vi "NANOTEC-MOTORS.vi"() -> ()   [LabVIEW 2013]
uses:
  global_notaus.vi
  global_log_file.vi
panel:
  out "Bool Ref":T1
  in  "Tab Control":T2(tab)=enum."Standard Motor Operation"
  out "Created New Semaphor":bool
  in  "ComPort (VISA in)":refnum<visa-resource-name>="COM1"
  in  "ComConfig":T3={"Baudrate (115200)"=115200, "Data Bits (8)"=8, "Parity (None)"=0, "Stop Bits (1)"=10, "Flow Control (None)"=0, "End Mode for Reads (TermChar)"=2} {"End Mode for Reads (TermChar)" items=["None", "Last Bit", "TermChar"]; "Flow Control (None)" items=["None", "XON/XOFF", "RTS/CTS", "XON/XOFF & RTS/CTS", "DTR/DSR", "XON/XOFF & DTR/DSR"]; "Stop Bits (1)" items=["1.0"=10, "1.5"=15, "2.0"=20]; "Parity (None)" items=["None", "Odd", "Even", "Mark", "Space"]; "Baudrate (115200)" items=["115200"=115200, "19200"=19200]}
  in  "error in (no error)":errorcluster
  in  "Firmware":bool
  in  "Error Reset":bool
  out "Firmware 2":string
  out "error out":errorcluster
  out "VISA ressource out":refnum<visa-resource-name>
  out "Answer to Command":string
  in  "Command":string
  in  "Send Command":bool
  out "Current Position 2":string
  in  "Motor Adress 1":T4(ring)=enum."3" caption="Motor Adress"
  out "Answer Save Profile":string
  out "Answer V Start":string
  out "Answer Ramp":string
  out "Answer Break":string
  out "Answer Direction":string
  out "Answer Steps":string
  in  "Direction (d)":i32(ring) items=["left", "right"]
  in  "Steps (s)":u32=400
  out "Answer Operation Mode":string
  in  "V Start (u)":u32=1
  in  "V Normal (o)":u32=400
  in  "Ramp (b)":u32=10
  in  "Break (B)":u32=10
  in  "Save Profile":bool
  out "Answer V Normal":string
  in  "Number of Profile (>)":u32=1
  in  "Operation Mode (p)":u16(ring)=1 items=["Relative Positioning"=1, "Absolute Positioning"=2, "Internal Reference"=3, "External Reference"=4, "Speed"=5]
  in  "Save and Drive Profile":bool
  in  "Current Position":bool
  in  "Drive Profile":bool
  in  "Start Profile":bool
  in  "Stop Profile":bool
  out "Answer Stop":string
  out "Answer Start":string
  in  "Load Profile":bool
  out "Answer Load Profile":string
  in  "Read Current Profile":bool
  out "Answer Read Current Profile":string
  in  "Profile Nr.":i32=123456
  in  "Motor Adress 2":T4(ring)=enum."3" caption="Motor Adress"
  out "Delta Steps":i32
  in  "steps 0":bool
  in  "Refresh Log File":bool
  in  "steps 60000":bool
  in  "steps 48000":bool
  in  "steps 10000":bool
  in  "steps 5000":bool
  in  "steps 1000":bool
  in  "steps 500":bool
  in  "steps 50":bool
  in  "steps 100":bool
  in  "steps master":i32
  in  "Reload Standard Pr Para":bool
  in  "Notaus":bool
  out "Log File 2":string
  in  "Delete Log File 2":bool
  in  "exp cclock":bool
  in  "exp clock":bool
  in  "prep cclock":bool
  in  "prep clock":bool
  in  "right":bool
  in  "left":bool
  in  "down":bool
  in  "up":bool
  in  "in":bool
  in  "out":bool
  in  "Save Waypoint":bool
  in  "Delete Log File":bool
  out "Log File":string
  in  "Waypoints":u16(ring)=1 items=["WP 1 "=1, "WP 2"=2, "WP 3"=3, "WP 4"=4, "WP 5"=5]
  in  "Go to Waypoint":bool
  in  "Test WP function":bool
  in  "Reload Waypoint Profiles from Save File":bool
  in  "Reload Drivers Digital Input":bool
  in  "stop":bool
  # "(leave out # and \\r)"
  # "(\"?\" means Command is invalid)"
  # "(in Hz)"
  # "(in Hz)"
  # "(in Hz/ms)"
  # "(in Hz/ms)"
  # "[1-32]"
  # "STEPS"
  # "Standard Profile Parameters for Operation of Motors (V_Start, V_Stop, Ramp, Break, etc.)\nfor this Tab can be manipulated in the Code (Event-Structure Frame 20)."
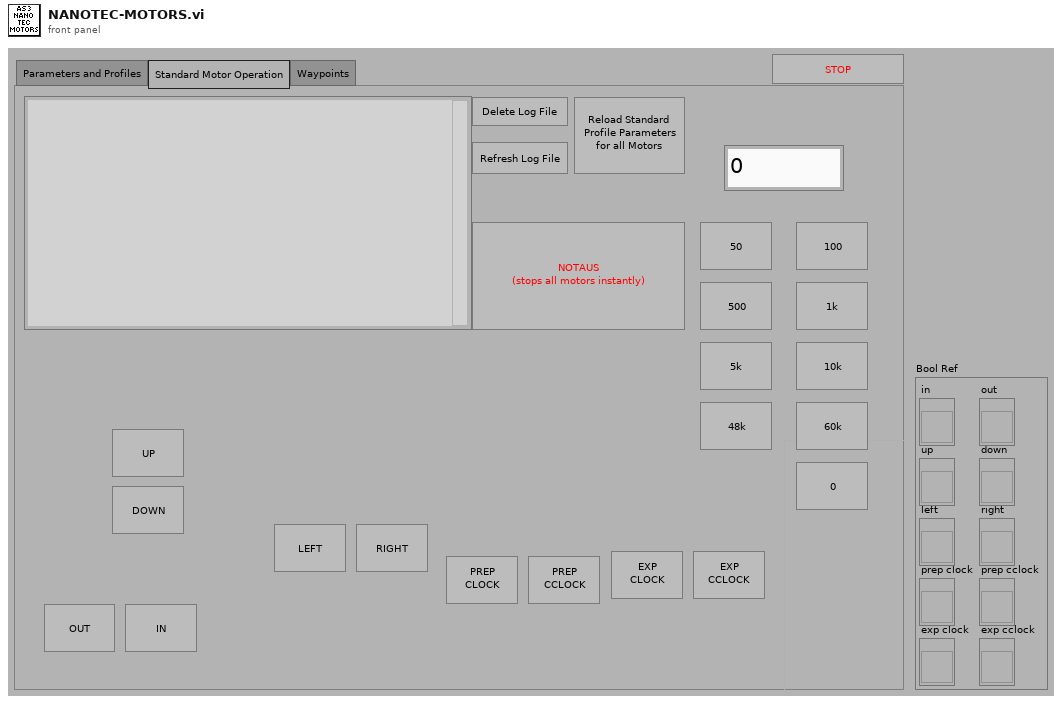
[diagram p1: front panel]
types:
  T1 = cluster{"in":refnum<vi>, "out":refnum<vi>, "up":refnum<vi>, "down":refnum<vi>, "left":refnum<vi>, "right":refnum<vi>, "prep clock":refnum<vi>, "prep cclock":refnum<vi>, "exp clock":refnum<vi>, "exp cclock":refnum<vi>}
  T2 = enum32{"Parameters and Profiles", "Standard Motor Operation", "Waypoints"}
  T3 = cluster{"Baudrate (115200)":u32, "Data Bits (8)":u16, "Parity (None)":u16, "Stop Bits (1)":u16, "Flow Control (None)":u16, "End Mode for Reads (TermChar)":u16}
  T4 = enum16{"All", "1", "2", "3", "4", "5", "6", "7", "8"}
  T5 = enum16{"open", "replace", "create", "open or create", "replace or create", "replace or create with confirmation"}
  T6 = typedef "Semaphore RefNum" = refnum<k1>
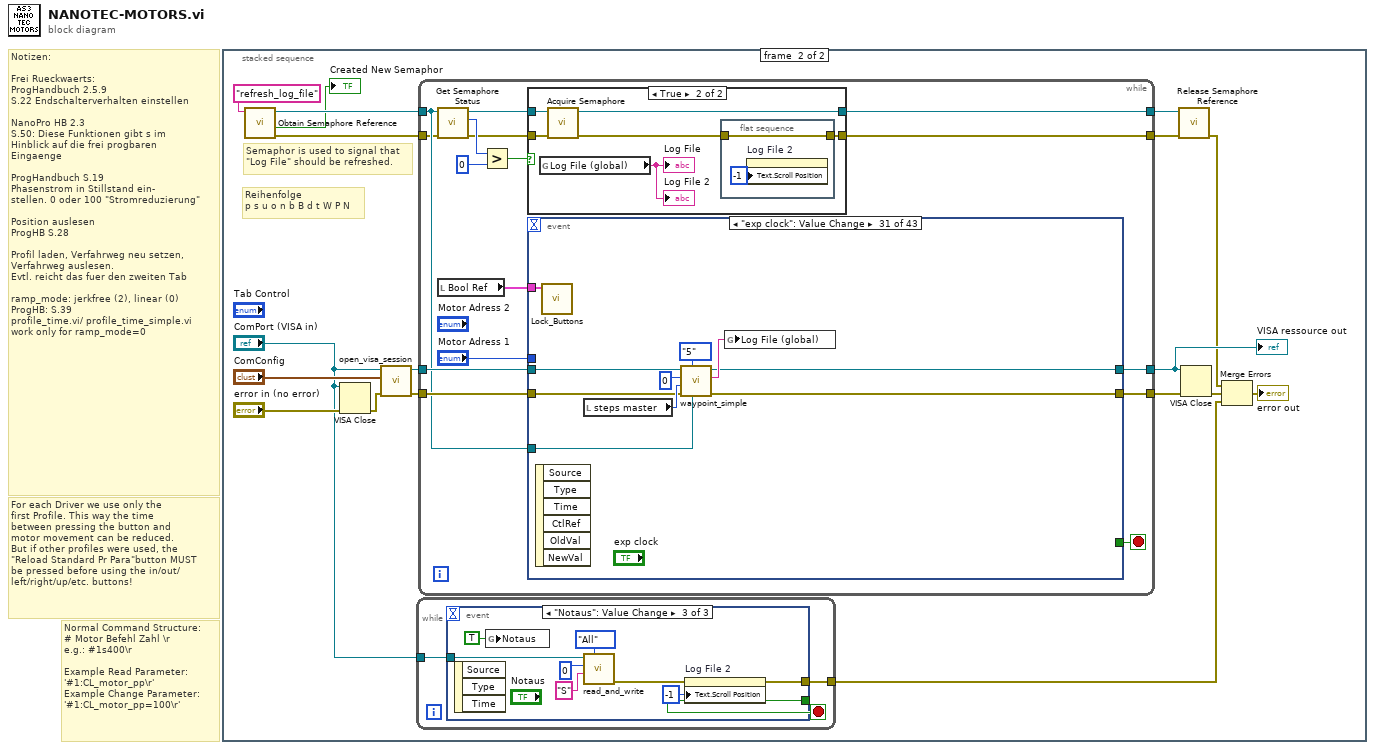
[diagram p0: block diagram]
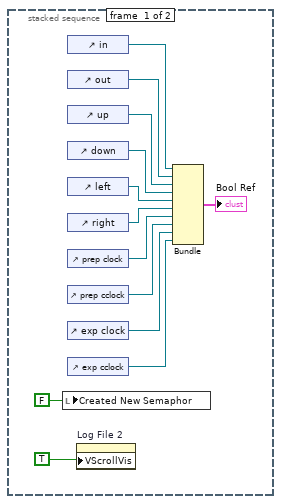
[diagram p2: hidden frame]
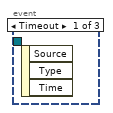
[diagram p3: hidden frame]
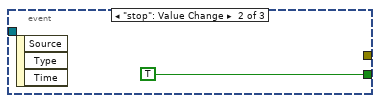
[diagram p4: hidden frame]
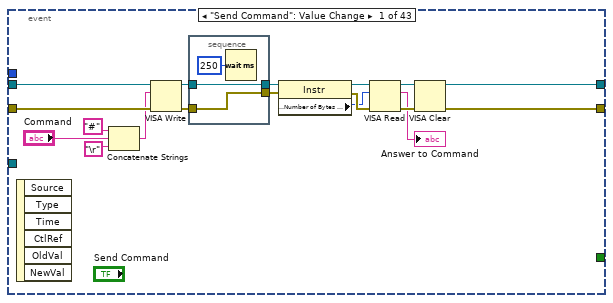
[diagram p6: hidden frame]
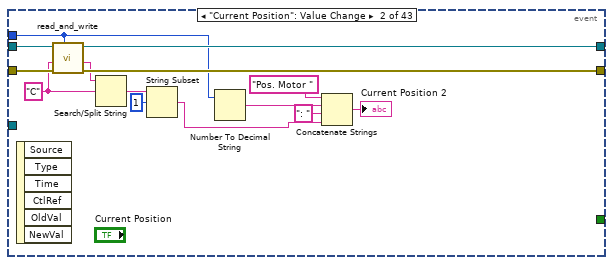
[diagram p7: hidden frame]
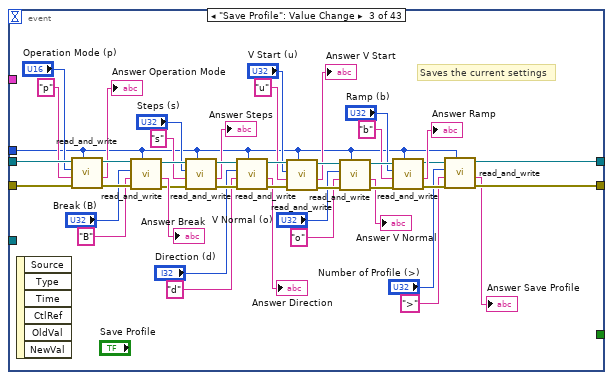
[diagram p8: hidden frame]
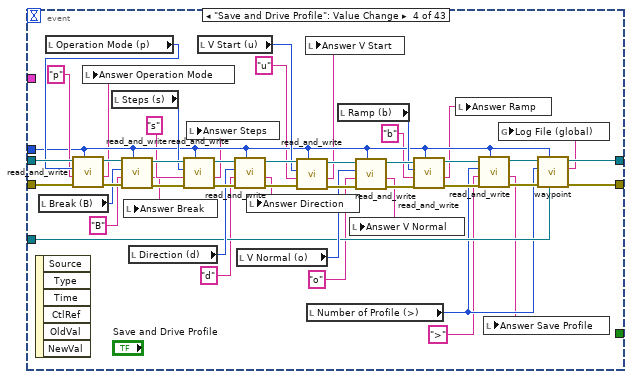
[diagram p9: hidden frame]
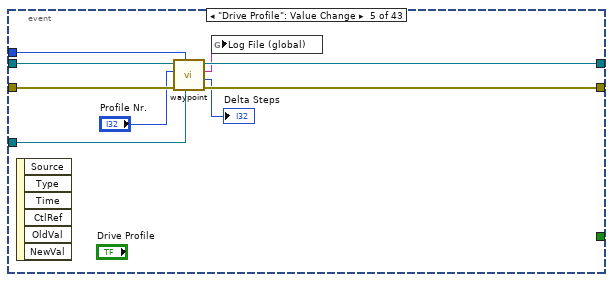
[diagram p10: hidden frame]
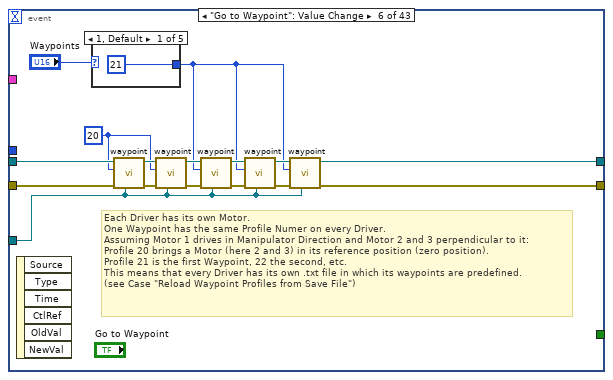
[diagram p11: hidden frame]
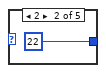
[diagram p12: hidden frame]
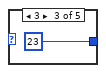
[diagram p13: hidden frame]
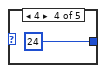
[diagram p14: hidden frame]
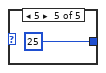
[diagram p15: hidden frame]
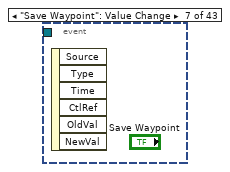
[diagram p16: hidden frame]
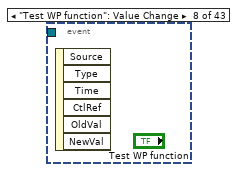
[diagram p17: hidden frame]
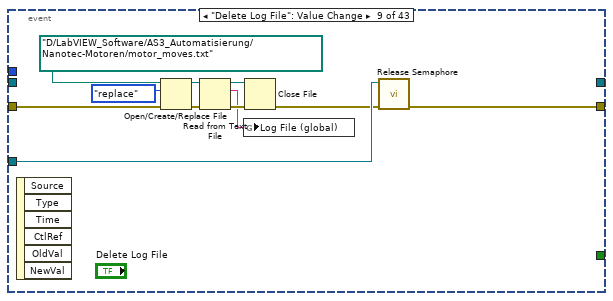
[diagram p18: hidden frame]
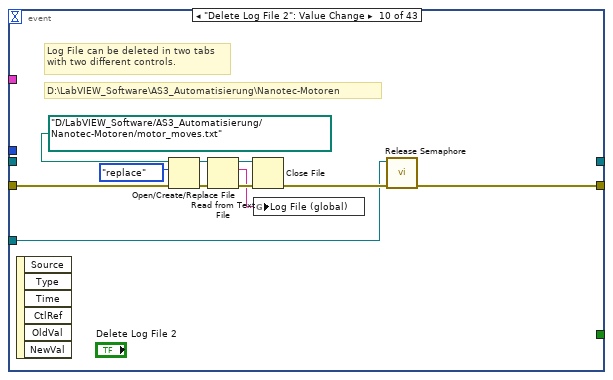
[diagram p19: hidden frame]
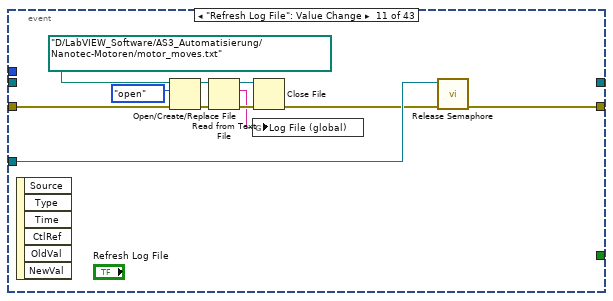
[diagram p20: hidden frame]
diagram:
  # "For each Driver we use only the\nfirst Profile. This way the time\nbetween pressing the button and\nmotor movement can be reduced.\nBut if other profiles were used, the\n\"Reload Standard Pr Para\"button MUST\nbe pressed before using the in/out/\nleft/right/up/etc. buttons!"
  # "Normal Command Structure:\n# Motor Befehl Zahl \\r\ne.g.: #1s400\\r\n\nExample Read Parameter:\n'#1:CL_motor_pp\\r'\nExample Change Parameter:\n'#1:CL_motor_pp=100\\r'"
  # "Notizen:\n\nFrei Rueckwaerts:\nProgHandbuch 2.5.9\nS.22 Endschalterverhalten einstellen\n\nNanoPro HB 2.3 \nS.50: Diese Funktionen gibt s im \nHinblick auf die frei progbaren \nEingaenge\n\nProgHandbuch S.19\nPhasenstrom in Stillstand ein-\nstellen. 0 oder 100 \"Stromreduzierung\"\n\nPosition auslesen\nProgHB S.28\n\nProfil laden, Verfahrweg neu setzen,\nVerfahrweg auslesen.\nEvtl. reicht das fuer den zweiten Tab\n\nramp_mode: jerkfree (2), linear (0) \nProgHB: S.39\nprofile_time.vi/ profile_time_simple.vi\nwork only for ramp_mode=0"
  n1 = stacked-sequence {
    frame #0 {
      n2 = local write "Created New Semaphor"(FALSE) -> ()
      n3 = control-ref of="in"() -> (w13:refnum<vi>)
      n4 = control-ref of="out"() -> (w12:refnum<vi>)
      n5 = control-ref of="up"() -> (w11:refnum<vi>)
      n6 = control-ref of="down"() -> (w10:refnum<vi>)
      n7 = control-ref of="left"() -> (w9:refnum<vi>)
      n8 = control-ref of="right"() -> (w8:refnum<vi>)
      n9 = control-ref of="prep clock"() -> (w7:refnum<vi>)
      n10 = control-ref of="prep cclock"() -> (w6:refnum<vi>)
      n11 = control-ref of="exp clock"() -> (w5:refnum<vi>)
      n12 = control-ref of="exp cclock"() -> (w4:refnum<vi>)
      n13 = property on="Log File 2" class="Str"("VScrollVis"=TRUE) -> ()  [unwired: 2 in, 2 out]
      n14 = Bundle("in"=w13, "out"=w12, "up"=w11, "down"=w10, "left"=w9, "right"=w8, "prep clock"=w7, "prep cclock"=w6, "exp clock"=w5, "exp cclock"=w4) -> (→"Bool Ref":T1)  [unwired: 1 in]
    }
    frame #1 {
      # "Reihenfolge\np s u o n b B d t W P N"
      # "Semaphor is used to signal that\n\"Log File\" should be refreshed."
      n15 = call <vilib>:"Obtain Semaphore Reference.vi"("name (unnamed)"="refresh_log_file") -> ("error out"=w21:errorcluster, "created new"=→"Created New Semaphor":bool, "semaphore"=w23:T6)  [unwired: 4 in]
      n16 = VISA Close(VISA resource name="ComPort (VISA in)", error in (no error)="error in (no error)") -> (error out=w27:errorcluster)
      n17 = call "open_visa_session.vi"("error in (no error)"=w27, "Cluster"="ComConfig", "ComPort"="ComPort (VISA in)") -> ("error out"=w30:errorcluster, "VISA resource name out"=w31:refnum<visa-resource-name>)  [unwired: 7 in]
      n18 = while {
        tunnel: "ComPort (VISA in)" -> [w33]
        tunnel: [w32] -> w14
        stop <- w34 stop-if-true
        n19 = event shown="[2] \"Notaus\": Value Change" {
          selector: _ -> [_ _ _]
          dyn-events: _ -> [_ _ _]
          timeout: _ -> [_ _ _]
          tunnel: [_ TRUE _] -> w34
          tunnel: w33 -> [_ _ w40]
          tunnel: [_ _ w36] -> w32
          event Timeout {
            n20 = event-data() -> ()  [unwired: 1 in, 3 out]
          }
          event "stop": Value Change {
            n21 = event-data() -> ()  [unwired: 1 in, 3 out]
          }
          event "Notaus": Value Change {
            n22 = event-data() -> ()  [unwired: 1 in, 3 out]
            n23 = global write "global_notaus.vi" "Notaus"(TRUE) -> ()
            n24 = call "read_and_write.vi"("Motor Adress"=T4."All", "Command"="S", "value"=0, "VISA ressource in"=w40) -> ("error out"=w37:errorcluster)  [unwired: 4 in, 3 out]
            n25 = property on="Log File 2" class="Str"(error in=w37, "Text.Scroll Position"=-1) -> (error out=w36:errorcluster)  [unwired: 1 in, 1 out]
          }
        }
      }
      n26 = while {
        tunnel: w31 -> [w59]
        tunnel: w30 -> [w58]
        tunnel: [w45] -> w29
        tunnel: [w57] -> w28
        tunnel: w23 -> [w50]
        tunnel: [w51] -> w22
        tunnel: w21 -> [w49]
        tunnel: [w47] -> w20
        stop <- w46 stop-if-true
        n27 = call <vilib>:"Get Semaphore Status.vi"("error in (no error)"=w49, "semaphore"=w50) -> ("error out"=w48:errorcluster, "# available"=w55:i32, "semaphore out"=w52:T6)  [unwired: 4 in, 3 out]
        n28 = local read "Bool Ref"() -> (w44:T1)
        n29 = Greater?(x=w55, y=0) -> (0:w53:bool)
        n30 = case shown="True" w53 {
          tunnel: w52 -> [w61 w67]
          tunnel: [w61 w66] -> w51
          tunnel: w48 -> [w60 w65]
          tunnel: [w60 w62] -> w47
          frame False {
          }
          frame True {
            n31 = global read "global_log_file.vi" "Log File (global)"() -> (→"Log File" →"Log File 2":string)
            n32 = call <vilib>:"Acquire Semaphore.vi"("error in (no error)"=w65, "semaphore"=w67) -> ("error out"=w63:errorcluster, "semaphore out"=w66:T6)  [unwired: 3 in, 1 out]
            n33 = flat-sequence {
              tunnel: w63 -> [w69]
              tunnel: [w69] -> w62
              frame #0 {
                n34 = property on="Log File 2" class="Str"("Text.Scroll Position"=-1) -> ()  [unwired: 2 in, 2 out]
              }
            }
          }
        }
        n35 = event shown="[30] \"exp clock\": Value Change" {
          selector: _ -> [_ _ _ _ _ _ _ _ _ _ _ _ _ _ _ _ _ _ _ _ _ _ _ _ _ _ _ _ _ _ _ _ _ _ _ _ _ _ _ _ _ _ _]
          dyn-events: _ -> [_ _ _ _ _ _ _ _ _ _ _ _ _ _ _ _ _ _ _ _ _ _ _ _ _ _ _ _ _ _ _ _ _ _ _ _ _ _ _ _ _ _ _]
          timeout: _ -> [_ _ _ _ _ _ _ _ _ _ _ _ _ _ _ _ _ _ _ _ _ _ _ _ _ _ _ _ _ _ _ _ _ _ _ _ _ _ _ _ _ _ _]
          tunnel: w59 -> [w78 w101 w146 w179 w203 w211 _ _ _ _ _ w265 w273 w281 w289 w294 w523 w575 w581 _ _ w587 w635 w643 w659 w669 w679 w689 w699 w709 w719 w729 _ _ _ _ _ _ _ _ _ _ _]
          tunnel: w58 -> [w77 w104 w147 w180 w202 w208 _ _ w232 w239 w249 w264 w272 w280 w288 w293 w521 w574 w580 _ _ w588 w633 w644 w653 w663 w673 w683 w693 w703 w713 w723 _ _ _ _ _ _ _ _ _ _ _]
          tunnel: [w76 w102 w124 w168 w201 w214 _ _ _ _ _ w261 w270 w279 w287 w291 w527 w572 w578 _ _ w585 w640 w647 w656 w666 w676 w686 w696 w706 w716 w726 _ _ _ _ _ _ _ _ _ _ _] -> w57
          tunnel: [w75 w103 w125 w166 w200 w215 _ _ w233 w237 w247 w260 w269 w278 w286 w292 w528 w571 w577 _ _ w586 w639 w648 w657 w667 w677 w687 w697 w707 w717 w727 _ _ _ _ _ _ _ _ _ _ _] -> w45
          tunnel: "Motor Adress 1" -> [_ w96 w105 w163 w199 _ _ _ _ _ _ w259 w267 w276 w283 w295 _ w569 w576 _ _ _ _ _ _ _ _ _ _ _ _ _ _ _ _ _ _ _ _ _ _ _ _]
          tunnel: w50 -> [_ _ _ w165 w197 w206 _ _ w234 w238 w257 _ _ w274 _ _ _ _ _ _ _ _ w637 w649 w658 w668 w678 w688 w698 w708 w718 w728 _ _ _ _ _ _ _ _ _ _ _]
          tunnel: [_ _ _ _ _ _ _ _ _ _ _ _ _ _ _ _ _ _ _ _ _ _ _ _ _ _ _ _ _ _ _ _ _ _ _ _ _ _ _ _ _ TRUE _] -> w46
          tunnel: w44 -> [_ _ _ _ _ _ _ _ _ _ _ _ _ _ _ _ _ _ _ _ _ _ w634 w645 w654 w664 w674 w684 w694 w704 w714 w724 _ _ _ _ _ _ _ _ _ _ _]
          event "Send Command": Value Change {
            n36 = event-data() -> ()  [unwired: 1 in, 6 out]
            n37 = Concatenate Strings("#" ("staticText"), "Command", "\r") -> (w72:string)
            n38 = VISA Write(VISA resource name=w78, write buffer=w72, error in (no error)=w77) -> (VISA resource name out=w82:refnum<visa-resource-name>, error out=w80:errorcluster)  [unwired: 1 out]
            n39 = stacked-sequence {
              tunnel: w82 -> [w90]
              tunnel: [w90] -> w81
              tunnel: w80 -> [w89]
              tunnel: [w89] -> w79
              frame #0 {
                n40 = Wait (ms)(milliseconds to wait=u32 250) -> ()  [unwired: 1 out]
              }
            }
            n41 = property class="Instr"(reference=w81, error in=w79) -> (reference out=w84:refnum<visa-resource-name>, error out=w85:errorcluster, "Serial Settings:Number of Bytes at Serial Port"=w83:u32)
            n42 = VISA Read(VISA resource name=w84, byte count=w83, error in (no error)=w85) -> (VISA resource name out=w87:refnum<visa-resource-name>, read buffer=→"Answer to Command":string, error out=w86:errorcluster)  [unwired: 1 out]
            n43 = VISA Clear(VISA resource name=w87, error in (no error)=w86) -> (VISA resource name out=w76:refnum<visa-resource-name>, error out=w75:errorcluster)
          }
          event "Current Position": Value Change {
            w99 = "C" ("Command")
            n44 = event-data() -> ()  [unwired: 1 in, 6 out]
            n45 = call "read_and_write.vi"("Motor Adress"=w96, "error in (no error)"=w104, "Command"=w99, "VISA ressource in"=w101) -> ("error out"=w103:errorcluster, "Answer"=w100:string, "VISA ressource out"=w102:refnum<visa-resource-name>)  [unwired: 4 in, 1 out]
            n46 = Search/Split String(string=w100, search string/char (-)=w99) -> (match + rest of string=w98:string)  [unwired: 1 in, 2 out]
            n47 = String Subset(string=w98, offset (0)=1) -> (substring=w91:string)  [unwired: 1 in]
            n48 = Number To Decimal String(number=w96) -> (decimal integer string=w94:string)  [unwired: 1 in]
            n49 = Concatenate Strings("Pos. Motor " ("string"), w94, ": " ("string"), w91) -> (→"Current Position 2":string)
          }
          event "Save Profile": Value Change {
            # "Saves the current settings"
            n50 = event-data() -> ()  [unwired: 1 in, 6 out]
            n51 = call "read_and_write.vi"("Motor Adress"=w105, "error in (no error)"=w147, "Command"="p" ("string"), "value"="Operation Mode (p)", "VISA ressource in"=w146) -> ("error out"=w144:errorcluster, "Answer"=→"Answer Operation Mode":string, "VISA ressource out"=w145:refnum<visa-resource-name>)  [unwired: 3 in, 1 out]
            n52 = call "read_and_write.vi"("Motor Adress"=w105, "error in (no error)"=w144, "Command"="B" ("command letter"), "value"="Break (B)", "VISA ressource in"=w145) -> ("error out"=w140:errorcluster, "Answer"=→"Answer Break":string, "VISA ressource out"=w141:refnum<visa-resource-name>)  [unwired: 3 in, 1 out]
            n53 = call "read_and_write.vi"("Motor Adress"=w105, "error in (no error)"=w140, "Command"="s" ("string"), "value"="Steps (s)", "VISA ressource in"=w141) -> ("error out"=w138:errorcluster, "Answer"=→"Answer Steps":string, "VISA ressource out"=w139:refnum<visa-resource-name>)  [unwired: 3 in, 1 out]
            n54 = call "read_and_write.vi"("Motor Adress"=w105, "error in (no error)"=w138, "Command"="d" ("string"), "value"="Direction (d)", "VISA ressource in"=w139) -> ("error out"=w136:errorcluster, "Answer"=→"Answer Direction":string, "VISA ressource out"=w137:refnum<visa-resource-name>)  [unwired: 3 in, 1 out]
            n55 = call "read_and_write.vi"("Motor Adress"=w105, "error in (no error)"=w136, "Command"="u" ("command letter"), "value"="V Start (u)", "VISA ressource in"=w137) -> ("error out"=w134:errorcluster, "Answer"=→"Answer V Start":string, "VISA ressource out"=w135:refnum<visa-resource-name>)  [unwired: 3 in, 1 out]
            n56 = call "read_and_write.vi"("Motor Adress"=w105, "error in (no error)"=w134, "Command"="o" ("command letter"), "value"="V Normal (o)", "VISA ressource in"=w135) -> ("error out"=w131:errorcluster, "Answer"=→"Answer V Normal":string, "VISA ressource out"=w129:refnum<visa-resource-name>)  [unwired: 3 in, 1 out]
            n57 = call "read_and_write.vi"("Motor Adress"=w105, "error in (no error)"=w131, "Command"="b" ("command letter"), "value"="Ramp (b)", "VISA ressource in"=w129) -> ("error out"=w127:errorcluster, "Answer"=→"Answer Ramp":string, "VISA ressource out"=w126:refnum<visa-resource-name>)  [unwired: 3 in, 1 out]
            n58 = call "read_and_write.vi"("Motor Adress"=w105, "error in (no error)"=w127, "Command"=">", "value"="Number of Profile (>)", "VISA ressource in"=w126) -> ("error out"=w125:errorcluster, "Answer"=→"Answer Save Profile":string, "VISA ressource out"=w124:refnum<visa-resource-name>)  [unwired: 3 in, 1 out]
          }
          event "Save and Drive Profile": Value Change {
            n59 = event-data() -> ()  [unwired: 1 in, 6 out]
            n60 = local read "Break (B)"() -> (w176:u32)
            n61 = local read "Operation Mode (p)"() -> (w178:u16)
            n62 = call "read_and_write.vi"("Motor Adress"=w163, "error in (no error)"=w180, "Command"="p", "value"=w178, "VISA ressource in"=w179) -> ("error out"=w193:errorcluster, "Answer"=w156:string, "VISA ressource out"=w194:refnum<visa-resource-name>)  [unwired: 3 in, 1 out]
            n63 = local write "Answer Operation Mode"(w156) -> ()
            n64 = local read "Steps (s)"() -> (w174:u32)
            n65 = call "read_and_write.vi"("Motor Adress"=w163, "error in (no error)"=w193, "Command"="B", "value"=w176, "VISA ressource in"=w194) -> ("error out"=w191:errorcluster, "Answer"=w155:string, "VISA ressource out"=w192:refnum<visa-resource-name>)  [unwired: 3 in, 1 out]
            n66 = local write "Answer Break"(w155) -> ()
            n67 = local read "Direction (d)"() -> (w173:i32)
            n68 = call "read_and_write.vi"("Motor Adress"=w163, "error in (no error)"=w191, "Command"="s", "value"=w174, "VISA ressource in"=w192) -> ("error out"=w189:errorcluster, "Answer"=w154:string, "VISA ressource out"=w190:refnum<visa-resource-name>)  [unwired: 3 in, 1 out]
            n69 = local write "Answer Steps"(w154) -> ()
            n70 = local read "V Start (u)"() -> (w172:u32)
            n71 = call "read_and_write.vi"("Motor Adress"=w163, "error in (no error)"=w189, "Command"="d", "value"=w173, "VISA ressource in"=w190) -> ("error out"=w187:errorcluster, "Answer"=w153:string, "VISA ressource out"=w188:refnum<visa-resource-name>)  [unwired: 3 in, 1 out]
            n72 = local read "V Normal (o)"() -> (w171:u32)
            n73 = local write "Answer Direction"(w153) -> ()
            n74 = call "read_and_write.vi"("Motor Adress"=w163, "error in (no error)"=w187, "Command"="u", "value"=w172, "VISA ressource in"=w188) -> ("error out"=w185:errorcluster, "Answer"=w152:string, "VISA ressource out"=w186:refnum<visa-resource-name>)  [unwired: 3 in, 1 out]
            n75 = local write "Answer V Start"(w152) -> ()
            n76 = local read "Number of Profile (>)"() -> (w164:u32)
            n77 = local read "Ramp (b)"() -> (w170:u32)
            n78 = call "read_and_write.vi"("Motor Adress"=w163, "error in (no error)"=w185, "Command"="o", "value"=w171, "VISA ressource in"=w186) -> ("error out"=w184:errorcluster, "Answer"=w151:string, "VISA ressource out"=w183:refnum<visa-resource-name>)  [unwired: 3 in, 1 out]
            n79 = local write "Answer V Normal"(w151) -> ()
            n80 = call "read_and_write.vi"("Motor Adress"=w163, "error in (no error)"=w184, "Command"="b", "value"=w170, "VISA ressource in"=w183) -> ("error out"=w182:errorcluster, "Answer"=w150:string, "VISA ressource out"=w181:refnum<visa-resource-name>)  [unwired: 3 in, 1 out]
            n81 = local write "Answer Ramp"(w150) -> ()
            n82 = call "read_and_write.vi"("Motor Adress"=w163, "error in (no error)"=w182, "Command"=">", "value"=w164, "VISA ressource in"=w181) -> ("error out"=w167:errorcluster, "Answer"=w149:string, "VISA ressource out"=w169:refnum<visa-resource-name>)  [unwired: 3 in, 1 out]
            n83 = local write "Answer Save Profile"(w149) -> ()
            n84 = call "waypoint.vi"("semaphore"=w165, "Motor Adress"=w163, "error in (no error)"=w167, "Profile Number"=w164, "VISA ressource in"=w169) -> ("error out"=w166:errorcluster, "Log File"=w148:string, "VISA ressource out"=w168:refnum<visa-resource-name>)  [unwired: 3 in, 1 out]
            n85 = global write "global_log_file.vi" "Log File (global)"(w148) -> ()
          }
          event "Drive Profile": Value Change {
            n86 = event-data() -> ()  [unwired: 1 in, 6 out]
            n87 = call "waypoint.vi"("semaphore"=w197, "Motor Adress"=w199, "error in (no error)"=w202, "Profile Number"="Profile Nr.", "VISA ressource in"=w203) -> ("error out"=w200:errorcluster, "Delta Steps"=→"Delta Steps":i32, "Log File"=w198:string, "VISA ressource out"=w201:refnum<visa-resource-name>)  [unwired: 3 in]
            n88 = global write "global_log_file.vi" "Log File (global)"(w198) -> ()
          }
          event "Go to Waypoint": Value Change {
            w204 = 20 ("Profile Number")
            # "Each Driver has its own Motor.\nOne Waypoint has the same Profile Numer on every Driver.\nAssuming Motor 1 drives in Manipulator Direction and Motor 2 and 3 perpendicular to it:\nProfile 20 brings a Motor (here 2 and 3) in its reference position (zero position).\nProfile 21 is the first Waypoint, 22 the second, etc.\nThis means that every Driver has its own .txt file in which its waypoints are predefined.\n(see Case \"Reload Waypoint Profiles from Save File\")"
            n89 = event-data() -> ()  [unwired: 1 in, 6 out]
            n90 = case shown="1, Default" "Waypoints" {
              tunnel: [21 22 23 24 25] -> w205
              frame 1, Default {
              }
              frame 2 {
              }
              frame 3 {
              }
              frame 4 {
              }
              frame 5 {
              }
            }
            n91 = call "waypoint.vi"("semaphore"=w206, "error in (no error)"=w208, "Profile Number"=w204, "VISA ressource in"=w211) -> ("error out"=w209:errorcluster, "VISA ressource out"=w212:refnum<visa-resource-name>)  [unwired: 4 in, 2 out]
            n92 = call "waypoint.vi"("semaphore"=w206, "error in (no error)"=w209, "Profile Number"=w204, "VISA ressource in"=w212) -> ("error out"=w207:errorcluster, "VISA ressource out"=w210:refnum<visa-resource-name>)  [unwired: 4 in, 2 out]
            n93 = call "waypoint.vi"("semaphore"=w206, "error in (no error)"=w207, "Profile Number"=w205, "VISA ressource in"=w210) -> ("error out"=w219:errorcluster, "VISA ressource out"=w218:refnum<visa-resource-name>)  [unwired: 4 in, 2 out]
            n94 = call "waypoint.vi"("semaphore"=w206, "error in (no error)"=w219, "Profile Number"=w205, "VISA ressource in"=w218) -> ("error out"=w217:errorcluster, "VISA ressource out"=w216:refnum<visa-resource-name>)  [unwired: 4 in, 2 out]
            n95 = call "waypoint.vi"("semaphore"=w206, "error in (no error)"=w217, "Profile Number"=w205, "VISA ressource in"=w216) -> ("error out"=w215:errorcluster, "VISA ressource out"=w214:refnum<visa-resource-name>)  [unwired: 4 in, 2 out]
          }
          event "Save Waypoint": Value Change {
            n96 = event-data() -> ()  [unwired: 1 in, 6 out]
          }
          event "Test WP function": Value Change {
            n97 = event-data() -> ()  [unwired: 1 in, 6 out]
          }
          event "Delete Log File": Value Change {
            n98 = event-data() -> ()  [unwired: 1 in, 6 out]
            n99 = Open/Create/Replace File(file path (use dialog)=path "D:/LabVIEW_Software/AS3_Automatisierung/Nanotec-Motoren/motor_moves.txt", error in=w232, operation (0:open)=T5."replace") -> (refnum out=w228:refnum<file>, error out=w230:errorcluster)  [unwired: 3 in, 1 out]
            n100 = Read from Text File(file (use dialog)=w228, error in=w230) -> (refnum out=w227:refnum<file>, text=w226:string, error out=w231:errorcluster)  [unwired: 2 in, 1 out]
            n101 = global write "global_log_file.vi" "Log File (global)"(w226) -> ()
            n102 = Close File(refnum=w227, error in=w231) -> (error out=w229:errorcluster)  [unwired: 1 out]
            n103 = call <vilib>:"Release Semaphore.vi"("error in (no error)"=w229, "semaphore"=w234) -> ("error out"=w233:errorcluster)  [unwired: 4 in, 1 out]
          }
          event "Delete Log File 2": Value Change {
            # "D:\\LabVIEW_Software\\AS3_Automatisierung\\Nanotec-Motoren"
            # "Log File can be deleted in two tabs\nwith two different controls."
            n104 = event-data() -> ()  [unwired: 1 in, 6 out]
            n105 = Open/Create/Replace File(file path (use dialog)=path "D:/LabVIEW_Software/AS3_Automatisierung/Nanotec-Motoren/motor_moves.txt", error in=w239, operation (0:open)=T5."replace") -> (refnum out=w242:refnum<file>, error out=w244:errorcluster)  [unwired: 3 in, 1 out]
            n106 = Read from Text File(file (use dialog)=w242, error in=w244) -> (refnum out=w241:refnum<file>, text=w240:string, error out=w245:errorcluster)  [unwired: 2 in, 1 out]
            n107 = Close File(refnum=w241, error in=w245) -> (error out=w243:errorcluster)  [unwired: 1 out]
            n108 = global write "global_log_file.vi" "Log File (global)"(w240) -> ()
            n109 = call <vilib>:"Release Semaphore.vi"("error in (no error)"=w243, "semaphore"=w238) -> ("error out"=w237:errorcluster)  [unwired: 4 in, 1 out]
          }
          event "Refresh Log File": Value Change {
            n110 = event-data() -> ()  [unwired: 1 in, 6 out]
            n111 = Open/Create/Replace File(file path (use dialog)=path "D:/LabVIEW_Software/AS3_Automatisierung/Nanotec-Motoren/motor_moves.txt", error in=w249, operation (0:open)=T5."open") -> (refnum out=w253:refnum<file>, error out=w254:errorcluster)  [unwired: 3 in, 1 out]
            n112 = Read from Text File(file (use dialog)=w253, error in=w254) -> (refnum out=w252:refnum<file>, text=w251:string, error out=w255:errorcluster)  [unwired: 2 in, 1 out]
            n113 = global write "global_log_file.vi" "Log File (global)"(w251) -> ()
            n114 = Close File(refnum=w252, error in=w255) -> (error out=w248:errorcluster)  [unwired: 1 out]
            n115 = call <vilib>:"Release Semaphore.vi"("error in (no error)"=w248, "semaphore"=w257) -> ("error out"=w247:errorcluster)  [unwired: 4 in, 1 out]
          }
          event "Load Profile": Value Change {
            n116 = event-data() -> ()  [unwired: 1 in, 6 out]
            n117 = local read "Profile Nr."() -> (w258:i32)
            n118 = call "read_and_write.vi"("Motor Adress"=w259, "error in (no error)"=w264, "Command"="y", "value"=w258, "VISA ressource in"=w265) -> ("error out"=w260:errorcluster, "Answer"=→"Answer Load Profile":string, "VISA ressource out"=w261:refnum<visa-resource-name>)  [unwired: 3 in, 1 out]
          }
          event "Read Current Profile": Value Change {
            n119 = event-data() -> ()  [unwired: 1 in, 6 out]
            n120 = call "read_and_write.vi"("additional waiting time"=u32 150, "Motor Adress"=w267, "error in (no error)"=w272, "Command"="Z|", "VISA ressource in"=w273) -> ("error out"=w269:errorcluster, "Answer"=→"Answer Read Current Profile":string, "VISA ressource out"=w270:refnum<visa-resource-name>)  [unwired: 3 in, 1 out]
          }
          event "Start Profile": Value Change {
            n121 = event-data() -> ()  [unwired: 1 in, 6 out]
            n122 = call "read_and_write.vi"("semaphore"=w274, "Motor Adress"=w276, "error in (no error)"=w280, "Command"="A", "VISA ressource in"=w281) -> ("error out"=w278:errorcluster, "Answer"=→"Answer Start":string, "Log File (global)"=w275:string, "VISA ressource out"=w279:refnum<visa-resource-name>)  [unwired: 3 in]
            n123 = global write "global_log_file.vi" "Log File (global)"(w275) -> ()
          }
          event "Stop Profile": Value Change {
            n124 = event-data() -> ()  [unwired: 1 in, 6 out]
            n125 = call "read_and_write.vi"("Motor Adress"=w283, "error in (no error)"=w288, "Command"="S", "value"=1, "VISA ressource in"=w289) -> ("error out"=w286:errorcluster, "Answer"=→"Answer Stop":string, "VISA ressource out"=w287:refnum<visa-resource-name>)  [unwired: 3 in, 1 out]
          }
          event "Reload Waypoint Profiles from Save File": Value Change {
            n126 = event-data() -> ()  [unwired: 1 in, 6 out]
            n127 = case shown="\"5\"" w295 {
              selector: w295 -> [w298 w321 w344 w365 w388 _ _ _ _]
              tunnel: w294 -> [w304 w327 w350 w366 w390 w412 w414 w416 w420]
              tunnel: w293 -> [w301 w324 w347 w367 w389 w411 w413 w415 w419]
              tunnel: [w303 w326 w349 w368 w392 w411 w413 w415 w418] -> w292
              tunnel: [w302 w325 w348 w369 w391 w412 w414 w416 w417] -> w291
              frame "1" {
                n128 = call "txt_to_array.vi"("error in"=w301, "file (use dialog)"=path "C:/Users/Admin/Desktop/AS3_Automatisierung/Nanotec-Motoren/WP_profiles_D1.txt") -> ("error out"=w300:errorcluster, "array"=w299:i32[][])  [unwired: 7 in, 1 out]
                n129 = for {
                  N: 6 -> [_]
                  tunnel: w304 -> [w318]
                  tunnel: w300 -> [w317]
                  tunnel: [w316] -> w303
                  tunnel: [w315] -> w302
                  tunnel: w299 -> [w314]
                  tunnel: w298 -> [w313]
                  i -> [w309]
                  n130 = Increment(x=w309) -> (x+1=w308:i32)
                  n131 = Array Subset(array=w314, index (row)=0 ("index"), length (row)=8 ("length"), index (col)=w308, length (col)=1 ("length")) -> (w307:i32[][])
                  n132 = Reshape Array(w307, 8 ("dimension size")) -> (w305:i32[])
                  n133 = call "save_profile.vi"("Motor Adress"=w313, "error in (no error)"=w317, "Profile Data"=w305, "VISA ressource in"=w318) -> ("error out"=w316:errorcluster, "VISA ressource out"=w315:refnum<visa-resource-name>)  [unwired: 6 in]
                }
              }
              frame "2" {
                n134 = call "txt_to_array.vi"("error in"=w324, "file (use dialog)"=path "C:/Users/Admin/Desktop/AS3_Automatisierung/Nanotec-Motoren/WP_profiles_D2.txt") -> ("error out"=w323:errorcluster, "array"=w322:i32[][])  [unwired: 7 in, 1 out]
                n135 = for {
                  N: 6 -> [_]
                  tunnel: w327 -> [w341]
                  tunnel: w323 -> [w340]
                  tunnel: [w339] -> w326
                  tunnel: [w338] -> w325
                  tunnel: w322 -> [w337]
                  tunnel: w321 -> [w336]
                  i -> [w332]
                  n136 = Increment(x=w332) -> (x+1=w331:i32)
                  n137 = Array Subset(array=w337, index (row)=0 ("index"), length (row)=8 ("length"), index (col)=w331, length (col)=1 ("length")) -> (w330:i32[][])
                  n138 = Reshape Array(w330, 8 ("dimension size")) -> (w328:i32[])
                  n139 = call "save_profile.vi"("Motor Adress"=w336, "error in (no error)"=w340, "Profile Data"=w328, "VISA ressource in"=w341) -> ("error out"=w339:errorcluster, "VISA ressource out"=w338:refnum<visa-resource-name>)  [unwired: 6 in]
                }
              }
              frame "3" {
                n140 = call "txt_to_array.vi"("error in"=w347, "file (use dialog)"=path "C:/Users/Admin/Desktop/AS3_Automatisierung/Nanotec-Motoren/WP_profiles_D3.txt") -> ("error out"=w346:errorcluster, "array"=w345:i32[][])  [unwired: 7 in, 1 out]
                n141 = for {
                  N: 6 -> [_]
                  tunnel: w350 -> [w364]
                  tunnel: w346 -> [w363]
                  tunnel: [w362] -> w349
                  tunnel: [w361] -> w348
                  tunnel: w345 -> [w360]
                  tunnel: w344 -> [w359]
                  i -> [w355]
                  n142 = Increment(x=w355) -> (x+1=w354:i32)
                  n143 = Array Subset(array=w360, index (row)=0 ("index"), length (row)=8 ("length"), index (col)=w354, length (col)=1 ("length")) -> (w353:i32[][])
                  n144 = Reshape Array(w353, 8 ("dimension size")) -> (w351:i32[])
                  n145 = call "save_profile.vi"("Motor Adress"=w359, "error in (no error)"=w363, "Profile Data"=w351, "VISA ressource in"=w364) -> ("error out"=w362:errorcluster, "VISA ressource out"=w361:refnum<visa-resource-name>)  [unwired: 6 in]
                }
              }
              frame "4" {
                n146 = call "txt_to_array.vi"("error in"=w367, "file (use dialog)"=path "C:/Users/Admin/Desktop/AS3_Automatisierung/Nanotec-Motoren/WP_profiles_D4.txt") -> ("error out"=w370:errorcluster, "array"=w371:i32[][])  [unwired: 7 in, 1 out]
                n147 = for {
                  N: 6 -> [_]
                  tunnel: w366 -> [w387]
                  tunnel: w370 -> [w386]
                  tunnel: [w385] -> w368
                  tunnel: [w384] -> w369
                  tunnel: w371 -> [w383]
                  tunnel: w365 -> [w382]
                  i -> [w378]
                  n148 = Increment(x=w378) -> (x+1=w377:i32)
                  n149 = Array Subset(array=w383, index (row)=0 ("index"), length (row)=8 ("length"), index (col)=w377, length (col)=1 ("length")) -> (w376:i32[][])
                  n150 = Reshape Array(w376, 8 ("dimension size")) -> (w374:i32[])
                  n151 = call "save_profile.vi"("Motor Adress"=w382, "error in (no error)"=w386, "Profile Data"=w374, "VISA ressource in"=w387) -> ("error out"=w385:errorcluster, "VISA ressource out"=w384:refnum<visa-resource-name>)  [unwired: 6 in]
                }
              }
              frame "5" {
                n152 = call "txt_to_array.vi"("error in"=w389, "file (use dialog)"=path "C:/Users/Admin/Desktop/AS3_Automatisierung/Nanotec-Motoren/WP_profiles_D5.txt") -> ("error out"=w393:errorcluster, "array"=w394:i32[][])  [unwired: 7 in, 1 out]
                n153 = for {
                  N: 6 -> [_]
                  tunnel: w390 -> [w410]
                  tunnel: w393 -> [w409]
                  tunnel: [w408] -> w392
                  tunnel: [w407] -> w391
                  tunnel: w394 -> [w406]
                  tunnel: w388 -> [w405]
                  i -> [w401]
                  n154 = Increment(x=w401) -> (x+1=w400:i32)
                  n155 = Array Subset(array=w406, index (row)=0 ("index"), length (row)=8 ("length"), index (col)=w400, length (col)=1 ("length")) -> (w399:i32[][])
                  n156 = Reshape Array(w399, 8 ("dimension size")) -> (w397:i32[])
                  n157 = call "save_profile.vi"("Motor Adress"=w405, "error in (no error)"=w409, "Profile Data"=w397, "VISA ressource in"=w410) -> ("error out"=w408:errorcluster, "VISA ressource out"=w407:refnum<visa-resource-name>)  [unwired: 6 in]
                }
              }
              frame "6" {
              }
              frame "7" {
              }
              frame "8" {
              }
              frame "All" {
                # "Lousy Error Handling, but code works either for all or none of the motors"
                n158 = stacked-sequence {
                  tunnel: w420 -> [w422 w441 w460 w479 w500]
                  tunnel: w419 -> [w421 w440 w459 w478 w499]
                  tunnel: [_ _ _ _ w497] -> w418
                  tunnel: [_ _ _ _ w498] -> w417
                  frame #0 {
                    n159 = call "txt_to_array.vi"("error in"=w421, "file (use dialog)"=path "D:/LabVIEW_Software/AS3_Automatisierung/Nanotec-Motoren/WP_profiles_D1.txt") -> ("error out"=w423:errorcluster, "array"=w424:i32[][])  [unwired: 7 in, 1 out]
                    n160 = for {
                      N: 6 -> [_]
                      tunnel: w422 -> [w439]
                      tunnel: w423 -> [w438]
                      tunnel: [w437] -> _
                      tunnel: [w436] -> _
                      tunnel: w424 -> [w435]
                      i -> [w431]
                      n161 = Increment(x=w431) -> (x+1=w430:i32)
                      n162 = Array Subset(array=w435, index (row)=0 ("index"), length (row)=8 ("length"), index (col)=w430, length (col)=1 ("length")) -> (w429:i32[][])
                      n163 = Reshape Array(w429, 8 ("dimension size")) -> (w427:i32[])
                      n164 = call "save_profile.vi"("error in (no error)"=w438, "Profile Data"=w427, "VISA ressource in"=w439) -> ("error out"=w437:errorcluster, "VISA ressource out"=w436:refnum<visa-resource-name>)  [unwired: 7 in]
                    }
                  }
                  frame #1 {
                    n165 = call "txt_to_array.vi"("error in"=w440, "file (use dialog)"=path "D:/LabVIEW_Software/AS3_Automatisierung/Nanotec-Motoren/WP_profiles_D2.txt") -> ("error out"=w442:errorcluster, "array"=w443:i32[][])  [unwired: 7 in, 1 out]
                    n166 = for {
                      N: 6 -> [_]
                      tunnel: w441 -> [w458]
                      tunnel: w442 -> [w457]
                      tunnel: [w456] -> _
                      tunnel: [w455] -> _
                      tunnel: w443 -> [w454]
                      i -> [w450]
                      n167 = Increment(x=w450) -> (x+1=w449:i32)
                      n168 = Array Subset(array=w454, index (row)=0 ("index"), length (row)=8 ("length"), index (col)=w449, length (col)=1 ("length")) -> (w448:i32[][])
                      n169 = Reshape Array(w448, 8 ("dimension size")) -> (w446:i32[])
                      n170 = call "save_profile.vi"("error in (no error)"=w457, "Profile Data"=w446, "VISA ressource in"=w458) -> ("error out"=w456:errorcluster, "VISA ressource out"=w455:refnum<visa-resource-name>)  [unwired: 7 in]
                    }
                  }
                  frame #2 {
                    n171 = call "txt_to_array.vi"("error in"=w459, "file (use dialog)"=path "D:/LabVIEW_Software/AS3_Automatisierung/Nanotec-Motoren/WP_profiles_D3.txt") -> ("error out"=w461:errorcluster, "array"=w462:i32[][])  [unwired: 7 in, 1 out]
                    n172 = for {
                      N: 6 -> [_]
                      tunnel: w460 -> [w477]
                      tunnel: w461 -> [w476]
                      tunnel: [w475] -> _
                      tunnel: [w474] -> _
                      tunnel: w462 -> [w473]
                      i -> [w469]
                      n173 = Increment(x=w469) -> (x+1=w468:i32)
                      n174 = Array Subset(array=w473, index (row)=0 ("index"), length (row)=8 ("length"), index (col)=w468, length (col)=1 ("length")) -> (w467:i32[][])
                      n175 = Reshape Array(w467, 8 ("dimension size")) -> (w465:i32[])
                      n176 = call "save_profile.vi"("error in (no error)"=w476, "Profile Data"=w465, "VISA ressource in"=w477) -> ("error out"=w475:errorcluster, "VISA ressource out"=w474:refnum<visa-resource-name>)  [unwired: 7 in]
                    }
                  }
                  frame #3 {
                    n177 = call "txt_to_array.vi"("error in"=w478, "file (use dialog)"=path "D:/LabVIEW_Software/AS3_Automatisierung/Nanotec-Motoren/WP_profiles_D4.txt") -> ("error out"=w480:errorcluster, "array"=w481:i32[][])  [unwired: 7 in, 1 out]
                    n178 = for {
                      N: 6 -> [_]
                      tunnel: w479 -> [w496]
                      tunnel: w480 -> [w495]
                      tunnel: [w494] -> _
                      tunnel: [w493] -> _
                      tunnel: w481 -> [w492]
                      i -> [w488]
                      n179 = Increment(x=w488) -> (x+1=w487:i32)
                      n180 = Array Subset(array=w492, index (row)=0 ("index"), length (row)=8 ("length"), index (col)=w487, length (col)=1 ("length")) -> (w486:i32[][])
                      n181 = Reshape Array(w486, 8 ("dimension size")) -> (w484:i32[])
                      n182 = call "save_profile.vi"("error in (no error)"=w495, "Profile Data"=w484, "VISA ressource in"=w496) -> ("error out"=w494:errorcluster, "VISA ressource out"=w493:refnum<visa-resource-name>)  [unwired: 7 in]
                    }
                  }
                  frame #4 {
                    n183 = call "txt_to_array.vi"("error in"=w499, "file (use dialog)"=path "D:/LabVIEW_Software/AS3_Automatisierung/Nanotec-Motoren/WP_profiles_D5.txt") -> ("error out"=w501:errorcluster, "array"=w502:i32[][])  [unwired: 7 in, 1 out]
                    n184 = for {
                      N: 6 -> [_]
                      tunnel: w500 -> [w517]
                      tunnel: w501 -> [w516]
                      tunnel: [w515] -> w497
                      tunnel: [w514] -> w498
                      tunnel: w502 -> [w513]
                      i -> [w509]
                      n185 = Increment(x=w509) -> (x+1=w508:i32)
                      n186 = Array Subset(array=w513, index (row)=0 ("index"), length (row)=8 ("length"), index (col)=w508, length (col)=1 ("length")) -> (w507:i32[][])
                      n187 = Reshape Array(w507, 8 ("dimension size")) -> (w505:i32[])
                      n188 = call "save_profile.vi"("error in (no error)"=w516, "Profile Data"=w505, "VISA ressource in"=w517) -> ("error out"=w515:errorcluster, "VISA ressource out"=w514:refnum<visa-resource-name>)  [unwired: 7 in]
                    }
                  }
                }
              }
            }
          }
          event "Reload Drivers Digital Input": Value Change {
            w524 = T4."3" ("Motor Adress")
            # "read funtion of port a: \":port_in_a\"\nset function of port a: \":port_in_a<number>\"\nFor <number> inputs \nsee Programmierhandbuch_V2.7.pdf page 31"
            n189 = event-data() -> ()  [unwired: 1 in, 6 out]
            n190 = call "read_and_write.vi"("error in (no error)"=w521, "Command"="l", "value"=5154, "VISA ressource in"=w523) -> ("error out"=w520:errorcluster, "VISA ressource out"=w522:refnum<visa-resource-name>)  [unwired: 4 in, 2 out]
            n191 = call "read_and_write.vi"("Motor Adress"=w524, "error in (no error)"=w520, "Command"=":port_in_a" ("string"), "value"=7, "VISA ressource in"=w522) -> ("error out"=w537:errorcluster, "VISA ressource out"=w533:refnum<visa-resource-name>)  [unwired: 3 in, 2 out]
            n192 = disable-structure shown="Deaktiviert" {
              disable-tunnel: w537 -> [w566 w567]
              disable-tunnel: ":port_in_b" ("command letter") -> [w561 _]
              disable-tunnel: ":port_in_c" ("command letter") -> [w559 _]
              disable-tunnel: w533 -> [w558 w568]
              disable-tunnel: ":port_in_d" ("command letter") -> [w552 _]
              disable-tunnel: ":port_in_e" ("command letter") -> [w551 _]
              disable-tunnel: ":port_in_f" ("command letter") -> [w550 _]
              disable-tunnel: ":port_in_g" ("command letter") -> [w549 _]
              disable-tunnel: [w548 w567] -> w528
              disable-tunnel: [w547 w568] -> w527
              disable-tunnel: ":port_in_h" ("command letter") -> [w546 _]
              disable-tunnel: w524 -> [w540 _]
              frame Disabled {
                n193 = call "read_and_write.vi"("Motor Adress"=w540, "error in (no error)"=w566, "Command"=w561, "value"=2, "VISA ressource in"=w558) -> ("error out"=w565:errorcluster, "VISA ressource out"=w557:refnum<visa-resource-name>)  [unwired: 3 in, 2 out]
                n194 = call "read_and_write.vi"("Motor Adress"=w540, "error in (no error)"=w565, "Command"=w559, "value"=3, "VISA ressource in"=w557) -> ("error out"=w560:errorcluster, "VISA ressource out"=w556:refnum<visa-resource-name>)  [unwired: 3 in, 2 out]
                n195 = call "read_and_write.vi"("Motor Adress"=w540, "error in (no error)"=w560, "Command"=w552, "value"=4, "VISA ressource in"=w556) -> ("error out"=w564:errorcluster, "VISA ressource out"=w555:refnum<visa-resource-name>)  [unwired: 3 in, 2 out]
                n196 = call "read_and_write.vi"("Motor Adress"=w540, "error in (no error)"=w564, "Command"=w551, "value"=5, "VISA ressource in"=w555) -> ("error out"=w563:errorcluster, "VISA ressource out"=w554:refnum<visa-resource-name>)  [unwired: 3 in, 2 out]
                n197 = call "read_and_write.vi"("Motor Adress"=w540, "error in (no error)"=w563, "Command"=w550, "value"=6, "VISA ressource in"=w554) -> ("error out"=w562:errorcluster, "VISA ressource out"=w553:refnum<visa-resource-name>)  [unwired: 3 in, 2 out]
                n198 = call "read_and_write.vi"("Motor Adress"=w540, "error in (no error)"=w562, "Command"=w549, "VISA ressource in"=w553) -> ("error out"=w539:errorcluster, "VISA ressource out"=w538:refnum<visa-resource-name>)  [unwired: 4 in, 2 out]
                n199 = call "read_and_write.vi"("Motor Adress"=w540, "error in (no error)"=w539, "Command"=w546, "VISA ressource in"=w538) -> ("error out"=w548:errorcluster, "VISA ressource out"=w547:refnum<visa-resource-name>)  [unwired: 4 in, 2 out]
              }
              frame Enabled {
              }
            }
          }
          event "Firmware": Value Change {
            n200 = event-data() -> ()  [unwired: 1 in, 6 out]
            n201 = call "read_and_write.vi"("Motor Adress"=w569, "error in (no error)"=w574, "Command"="v", "VISA ressource in"=w575) -> ("error out"=w571:errorcluster, "Answer"=→"Firmware 2":string, "VISA ressource out"=w572:refnum<visa-resource-name>)  [unwired: 4 in, 1 out]
          }
          event "Error Reset": Value Change {
            n202 = event-data() -> ()  [unwired: 1 in, 6 out]
            n203 = call "read_and_write.vi"("Motor Adress"=w576, "error in (no error)"=w580, "Command"="D0", "VISA ressource in"=w581) -> ("error out"=w577:errorcluster, "VISA ressource out"=w578:refnum<visa-resource-name>)  [unwired: 4 in, 2 out]
          }
          event "Motor Adress 1": Value Change {
            n204 = event-data() -> ()  [unwired: 1 in, 6 out]
            n205 = local read "Motor Adress 1"() -> (w582:T4)
            n206 = local write "Motor Adress 2"(w582) -> ()
          }
          event "Motor Adress 2": Value Change {
            n207 = event-data() -> ()  [unwired: 1 in, 6 out]
            n208 = local read "Motor Adress 2"() -> (w583:T4)
            n209 = local write "Motor Adress 1"(w583) -> ()
          }
          event "Reload Standard Pr Para": Value Change {
            # "Reihenfolge fuer Array p B s u o b d >\np=1 (positioning mode)  B=10 (Break acceleration) \ns=1 (number of steps; will be changed by input anyway) \nu=1 (starting frequency)  o=400 (normal/ driving frequency)\nb=10 (Ramp acceleration)  d=0/1 (direction; changed by input as well)\n>=1/2 (Number of Profile)"
            n210 = event-data() -> ()  [unwired: 1 in, 6 out]
            n211 = for {
              N: 5 -> [_]
              tunnel: w588 -> [w597]
              tunnel: w587 -> [w596]
              tunnel: [w595] -> w586
              tunnel: [w594] -> w585
              i -> [w590]
              n212 = Increment(x=w590) -> (x+1=w589:i32)
              n213 = case shown="1, Default" w589 {
                tunnel: [T4."1" ("Motor Adress") T4."2" ("Motor Adress") T4."3" ("Motor Adress") T4."4" ("Motor Adress") T4."5" ("Motor Adress")] -> w593
                tunnel: [w603 w610 w617 w624 w631] -> w592
                frame 1, Default {
                  w600 = 10.0 ("Element")
                  w602 = 1.0 ("Element")
                  n214 = Build Array(w602, w600, w602, w602, 550.0 ("Element"), w600, 0.0 ("Element"), 1.0 ("Element")) -> (w603:dbl[])
                }
                frame 2 {
                  w607 = 10.0 ("Element")
                  w609 = 1.0 ("Element")
                  n215 = Build Array(w609, w607, w609, w609, 550.0 ("Element"), w607, 0.0 ("Element"), 1.0 ("Element")) -> (w610:dbl[])
                }
                frame 3 {
                  w614 = 10.0 ("Element")
                  w616 = 1.0 ("Element")
                  n216 = Build Array(w616, w614, w616, w616, 550.0 ("Element"), w614, 0.0 ("Element"), 1.0 ("Element")) -> (w617:dbl[])
                }
                frame 4 {
                  w621 = 10.0 ("Element")
                  w623 = 1.0 ("Element")
                  n217 = Build Array(w623, w621, w623, w623, 550.0 ("Element"), w621, 0.0 ("Element"), 1.0 ("Element")) -> (w624:dbl[])
                }
                frame 5 {
                  w628 = 10.0 ("Element")
                  w630 = 1.0 ("Element")
                  n218 = Build Array(w630, w628, w630, w630, 550.0 ("Element"), w628, 0.0 ("Element"), 1.0 ("Element")) -> (w631:dbl[])
                }
              }
              n219 = To Long Integer(number=w592) -> (32bit integer=w591:i32[])
              n220 = call "save_profile.vi"("Motor Adress"=w593, "error in (no error)"=w597, "Profile Data"=w591, "VISA ressource in"=w596) -> ("error out"=w595:errorcluster, "VISA ressource out"=w594:refnum<visa-resource-name>)  [unwired: 6 in]
            }
          }
          event "in": Value Change {
            # "left 0     profile 1\nright 1  profile 2"
            n221 = event-data() -> ()  [unwired: 1 in, 6 out]
            n222 = call "Lock_Buttons.vi"("Bool Reference"=w634) -> ()  [unwired: 10 in, 1 out]
            n223 = call "waypoint_simple.vi"("semaphore"=w637, "Motor Adress"=T4."1", "error in (no error)"=w633, "steps"="steps master", "Direction (d)"=1 ("Profile Number"), "VISA ressource in"=w635) -> ("error out"=w639:errorcluster, "Log File"=w638:string, "VISA ressource out"=w640:refnum<visa-resource-name>)  [unwired: 2 in, 1 out]
            n224 = global write "global_log_file.vi" "Log File (global)"(w638) -> ()
          }
          event "out": Value Change {
            n225 = event-data() -> ()  [unwired: 1 in, 6 out]
            n226 = call "Lock_Buttons.vi"("Bool Reference"=w645) -> ()  [unwired: 10 in, 1 out]
            n227 = local read "steps master"() -> (w646:i32)
            n228 = call "waypoint_simple.vi"("semaphore"=w649, "Motor Adress"=T4."1", "error in (no error)"=w644, "steps"=w646, "Direction (d)"=0 ("Profile Number"), "VISA ressource in"=w643) -> ("error out"=w648:errorcluster, "Log File"=w652:string, "VISA ressource out"=w647:refnum<visa-resource-name>)  [unwired: 2 in, 1 out]
            n229 = global write "global_log_file.vi" "Log File (global)"(w652) -> ()
          }
          event "up": Value Change {
            n230 = event-data() -> ()  [unwired: 1 in, 6 out]
            n231 = call "Lock_Buttons.vi"("Bool Reference"=w654) -> ()  [unwired: 10 in, 1 out]
            n232 = local read "steps master"() -> (w655:i32)
            n233 = call "waypoint_simple.vi"("semaphore"=w658, "Motor Adress"=T4."2", "error in (no error)"=w653, "steps"=w655, "Direction (d)"=0 ("Profile Number"), "VISA ressource in"=w659) -> ("error out"=w657:errorcluster, "Log File"=w662:string, "VISA ressource out"=w656:refnum<visa-resource-name>)  [unwired: 2 in, 1 out]
            n234 = global write "global_log_file.vi" "Log File (global)"(w662) -> ()
          }
          event "down": Value Change {
            n235 = event-data() -> ()  [unwired: 1 in, 6 out]
            n236 = call "Lock_Buttons.vi"("Bool Reference"=w664) -> ()  [unwired: 10 in, 1 out]
            n237 = local read "steps master"() -> (w665:i32)
            n238 = call "waypoint_simple.vi"("semaphore"=w668, "Motor Adress"=T4."2", "error in (no error)"=w663, "steps"=w665, "Direction (d)"=1 ("Profile Number"), "VISA ressource in"=w669) -> ("error out"=w667:errorcluster, "Log File"=w672:string, "VISA ressource out"=w666:refnum<visa-resource-name>)  [unwired: 2 in, 1 out]
            n239 = global write "global_log_file.vi" "Log File (global)"(w672) -> ()
          }
          event "left": Value Change {
            n240 = event-data() -> ()  [unwired: 1 in, 6 out]
            n241 = call "Lock_Buttons.vi"("Bool Reference"=w674) -> ()  [unwired: 10 in, 1 out]
            n242 = local read "steps master"() -> (w675:i32)
            n243 = call "waypoint_simple.vi"("semaphore"=w678, "Motor Adress"=T4."3", "error in (no error)"=w673, "steps"=w675, "Direction (d)"=1 ("Profile Number"), "VISA ressource in"=w679) -> ("error out"=w677:errorcluster, "Log File"=w682:string, "VISA ressource out"=w676:refnum<visa-resource-name>)  [unwired: 2 in, 1 out]
            n244 = global write "global_log_file.vi" "Log File (global)"(w682) -> ()
          }
          event "right": Value Change {
            n245 = event-data() -> ()  [unwired: 1 in, 6 out]
            n246 = call "Lock_Buttons.vi"("Bool Reference"=w684) -> ()  [unwired: 10 in, 1 out]
            n247 = local read "steps master"() -> (w685:i32)
            n248 = call "waypoint_simple.vi"("semaphore"=w688, "Motor Adress"=T4."3", "error in (no error)"=w683, "steps"=w685, "Direction (d)"=0 ("Profile Number"), "VISA ressource in"=w689) -> ("error out"=w687:errorcluster, "Log File"=w692:string, "VISA ressource out"=w686:refnum<visa-resource-name>)  [unwired: 2 in, 1 out]
            n249 = global write "global_log_file.vi" "Log File (global)"(w692) -> ()
          }
          event "prep clock": Value Change {
            n250 = event-data() -> ()  [unwired: 1 in, 6 out]
            n251 = call "Lock_Buttons.vi"("Bool Reference"=w694) -> ()  [unwired: 10 in, 1 out]
            n252 = local read "steps master"() -> (w695:i32)
            n253 = call "waypoint_simple.vi"("semaphore"=w698, "Motor Adress"=T4."4", "error in (no error)"=w693, "steps"=w695, "Direction (d)"=0 ("Profile Number"), "VISA ressource in"=w699) -> ("error out"=w697:errorcluster, "Log File"=w702:string, "VISA ressource out"=w696:refnum<visa-resource-name>)  [unwired: 2 in, 1 out]
            n254 = global write "global_log_file.vi" "Log File (global)"(w702) -> ()
          }
          event "prep cclock": Value Change {
            n255 = event-data() -> ()  [unwired: 1 in, 6 out]
            n256 = call "Lock_Buttons.vi"("Bool Reference"=w704) -> ()  [unwired: 10 in, 1 out]
            n257 = local read "steps master"() -> (w705:i32)
            n258 = call "waypoint_simple.vi"("semaphore"=w708, "Motor Adress"=T4."4", "error in (no error)"=w703, "steps"=w705, "Direction (d)"=1 ("Profile Number"), "VISA ressource in"=w709) -> ("error out"=w707:errorcluster, "Log File"=w712:string, "VISA ressource out"=w706:refnum<visa-resource-name>)  [unwired: 2 in, 1 out]
            n259 = global write "global_log_file.vi" "Log File (global)"(w712) -> ()
          }
          event "exp clock": Value Change {
            n260 = event-data() -> ()  [unwired: 1 in, 6 out]
            n261 = call "Lock_Buttons.vi"("Bool Reference"=w714) -> ()  [unwired: 10 in, 1 out]
            n262 = local read "steps master"() -> (w715:i32)
            n263 = call "waypoint_simple.vi"("semaphore"=w718, "Motor Adress"=T4."5", "error in (no error)"=w713, "steps"=w715, "Direction (d)"=0 ("Profile Number"), "VISA ressource in"=w719) -> ("error out"=w717:errorcluster, "Log File"=w722:string, "VISA ressource out"=w716:refnum<visa-resource-name>)  [unwired: 2 in, 1 out]
            n264 = global write "global_log_file.vi" "Log File (global)"(w722) -> ()
          }
          event "exp cclock": Value Change {
            n265 = event-data() -> ()  [unwired: 1 in, 6 out]
            n266 = call "Lock_Buttons.vi"("Bool Reference"=w724) -> ()  [unwired: 10 in, 1 out]
            n267 = local read "steps master"() -> (w725:i32)
            n268 = call "waypoint_simple.vi"("semaphore"=w728, "Motor Adress"=T4."5", "error in (no error)"=w723, "steps"=w725, "Direction (d)"=1 ("Profile Number"), "VISA ressource in"=w729) -> ("error out"=w727:errorcluster, "Log File"=w732:string, "VISA ressource out"=w726:refnum<visa-resource-name>)  [unwired: 2 in, 1 out]
            n269 = global write "global_log_file.vi" "Log File (global)"(w732) -> ()
          }
          event "steps 0": Value Change {
            n270 = event-data() -> ()  [unwired: 1 in, 6 out]
            n271 = local write "steps master"(0) -> ()
          }
          event "steps 50": Value Change {
            n272 = event-data() -> ()  [unwired: 1 in, 6 out]
            n273 = local write "steps master"(50) -> ()
          }
          event "steps 100": Value Change {
            n274 = event-data() -> ()  [unwired: 1 in, 6 out]
            n275 = local write "steps master"(100) -> ()
          }
          event "steps 500": Value Change {
            n276 = event-data() -> ()  [unwired: 1 in, 6 out]
            n277 = local write "steps master"(500) -> ()
          }
          event "steps 1000": Value Change {
            n278 = event-data() -> ()  [unwired: 1 in, 6 out]
            n279 = local write "steps master"(1000) -> ()
          }
          event "steps 5000": Value Change {
            n280 = event-data() -> ()  [unwired: 1 in, 6 out]
            n281 = local write "steps master"(5000) -> ()
          }
          event "steps 10000": Value Change {
            n282 = event-data() -> ()  [unwired: 1 in, 6 out]
            n283 = local write "steps master"(10000) -> ()
          }
          event "steps 48000": Value Change {
            n284 = event-data() -> ()  [unwired: 1 in, 6 out]
            n285 = local write "steps master"(48000) -> ()
          }
          event "steps 60000": Value Change {
            n286 = event-data() -> ()  [unwired: 1 in, 6 out]
            n287 = local write "steps master"(60000) -> ()
          }
          event "stop": Value Change {
            n288 = event-data() -> ()  [unwired: 1 in, 6 out]
          }
          event Timeout {
            n289 = event-data() -> ()  [unwired: 1 in, 2 out]
          }
        }
      }
      "VISA ressource out" <- w28
      n290 = call <vilib>:"Release Semaphore Reference.vi"("error in (no error)"=w20, "semaphore"=w22) -> ("error out"=w17:errorcluster)  [unwired: 8 in, 1 out]
      n291 = VISA Close(VISA resource name=w28, error in (no error)=w29) -> (error out=w19:errorcluster)
      n292 = Merge Errors(w17, w19, w14) -> (→"error out":errorcluster)
    }
  }
